vi "niFpga wdp fft streaming control chain dummy.vi"(6 "enable":bool, 8 "enable 1":bool, 11 "input frame start":bool) -> (0 "frame start":bool, 1 "index=0?":bool, 2 "switch":bool[](array[boolean]), 3 "twiddle factors 1":T1(array[cluster]), 5 "twiddle factors":T1(array[cluster]))   [LabVIEW 2017]
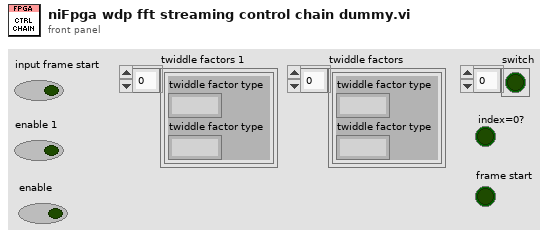
[diagram p1: front panel]
types:
  T1 = cluster{"twiddle factor type":fxp<+/-,16,2>, "twiddle factor type":fxp<+/-,16,2>}[]
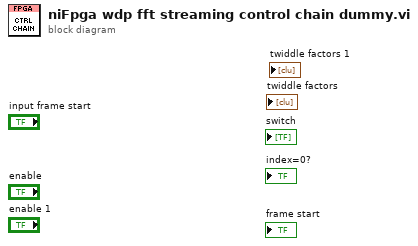
[diagram p0: block diagram]
diagram:
